vi "vectorProperties.vi"(10 "Goal \nplatform":i32, 11 "Start \nplatform":i32) -> (2 "vector \nangle":dbl, 3 "vector length":dbl)   [LabVIEW 2017]
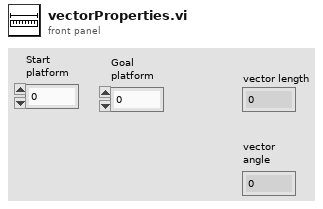
[diagram p1: front panel]
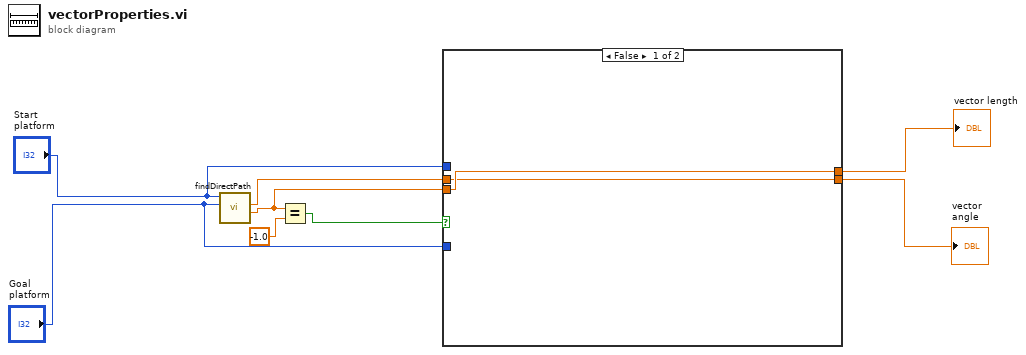
[diagram p0: block diagram]
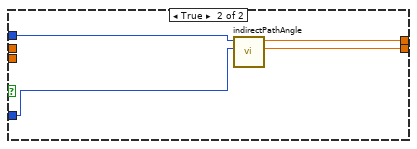
[diagram p2: hidden frame]
diagram:
  n1 = call "findDirectPath.vi"("goal platform"="Goal \nplatform", "start platform"="Start \nplatform") -> ("vector \nlength"=w2:dbl, "vector\nangle"=w1:dbl)  [unwired: 6 in, 2 out]
  n2 = Equal?(x=w2, y=-1.0) -> (x = y?=w5:bool)
  n3 = case shown="False" w5 {
    tunnel: "Start \nplatform" -> [_ w14]
    tunnel: "Goal \nplatform" -> [_ w13]
    tunnel: [w10 w12] -> w4
    tunnel: [w9 w11] -> w3
    tunnel: w2 -> [w10 _]
    tunnel: w1 -> [w9 _]
    frame False {
    }
    frame True {
      n4 = call "indirectPathAngle.vi"("goal platform"=w13, "start platform"=w14) -> ("vector \nangle"=w11:dbl, "vector length"=w12:dbl)  [unwired: 8 in]
    }
  }
  "vector length" <- w4
  "vector \nangle" <- w3
